vi "LNLS Control Saturation minus10 10.vi"(11 "in":dbl) -> (3 "saturated out":dbl)   [LabVIEW 2011, in "LNLS Control VIs.lvlib"]
uses:
  LNLS Control VIs.lvlib
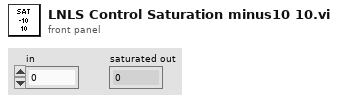
[diagram p1: front panel]
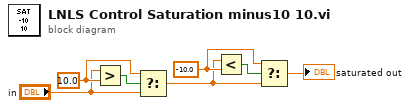
[diagram p0: block diagram]
diagram:
  w6 = 10.0
  w5 = -10.0
  n1 = Greater?(x="in", y=w6) -> (0:w3:bool)
  n2 = Select(t=w6, s=w3, f="in") -> (s? t:f=w1:dbl)
  n3 = Less?(x=w1, y=w5) -> (x < y?=w4:bool)
  n4 = Select(t=w5, s=w4, f=w1) -> (s? t:f=→"saturated out":dbl)
